vi "Move piezo.vi"(7 "error in (no error)":errorcluster, 8 "MOVE TO [MICRON]":dbl=1.0 format="%0.2f", 9 "notifier out":refnum<notifier>, 10 "Hardware Config In":T1={"physical channels"="Dev4/ao0", "MAX   VOLTAGE"=10.0, "MIN   VOLTAGE"=0.0}) -> (0 "error out":errorcluster, 3 "Hardware Config Out":T1={"physical channels"="Dev4/ao0", "MAX   VOLTAGE"=10.0, "MIN   VOLTAGE"=0.0})   [LabVIEW 2013, in "Piezo.lvlib"]
uses:
  Piezo/Piezo.lvlib
  Piezo/Piezo display.ctl
  Untitled Project 3 Andrea/piezo new/Hardware Configuration Piezo out.ctl
  <vilib>/DAQmx/write.llb/DAQmx Write (Analog DBL 1Chan 1Samp).vi
  <vilib>/DAQmx/create/channels.llb/DAQmx Create Channel (AO-Voltage-Basic).vi
  <vilib>/DAQmx/miscellaneous.llb/DAQmx Fill In Error Info.vi
panel:
  out "PiezoPosition":sgl
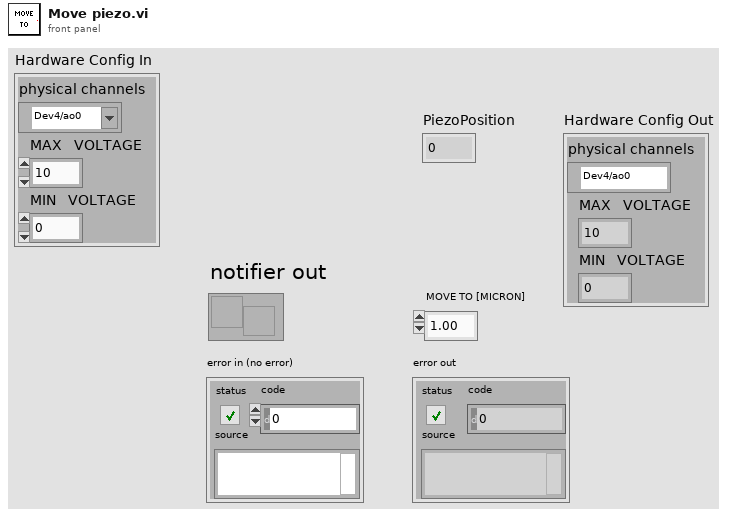
[diagram p1: front panel]
types:
  T1 = typedef "Hardware Configuration Piezo out.ctl" = cluster{"physical channels":tag, "MAX   VOLTAGE":dbl, "MIN   VOLTAGE":dbl}
  T2 = typedef "Piezo.lvlib/Piezo display.ctl" = cluster{"PiezoPosition":sgl, "Counter Time":i32}
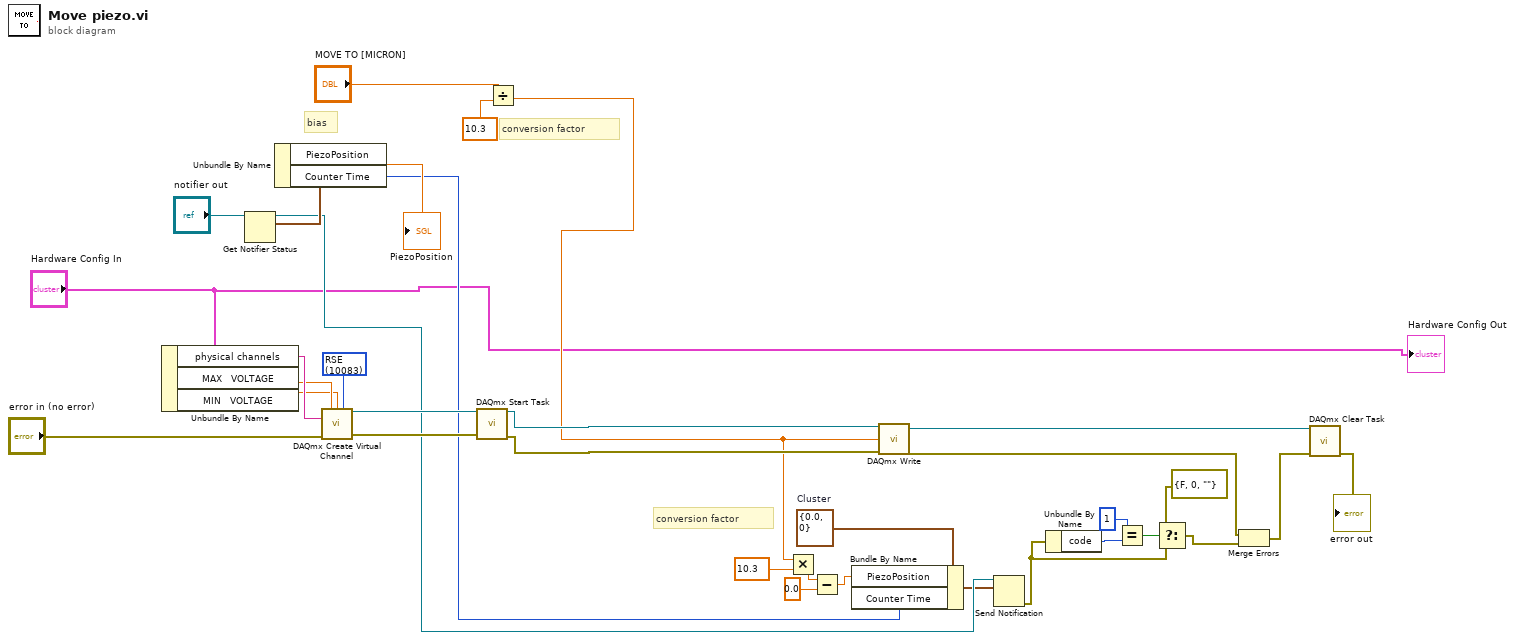
[diagram p0: block diagram]
diagram:
  w14 = T2 {"PiezoPosition"=0.0, "Counter Time"=0}  # Cluster
  w30 = 10083 items=["Default"=-1, "RSE"=10083, "Differential"=10106, "Pseudodifferential"=12529] ("output terminal configuration")
  # "conversion factor"
  # "bias"
  # "conversion factor"
  n1 = Unbundle By Name("Hardware Config In") -> ("physical channels"=w27:tag, "MAX   VOLTAGE"=w26:dbl, "MIN   VOLTAGE"=w25:dbl)
  n2 = Get Notifier Status(notifier="notifier out") -> (notifier out=w18:refnum<notifier>, current notification=w32:T2)  [unwired: 1 in, 3 out]
  n3 = Unbundle By Name(w32) -> ("PiezoPosition"=→"PiezoPosition":sgl, "Counter Time"=w17:i32)
  n4 = call-poly <vilib>:"DAQmx Create Virtual Channel.vi"("maximum value"=w26, "minimum value"=w25, "output terminal configuration"=w30, "physical channels"=w27, "error in"="error in (no error)") -> ("task out"=w29:refnum<k21>, "error out"=w28:errorcluster)  [unwired: 9 in]
  n5 = call <vilib>:"DAQmx Start Task.vi"("task/channels in"=w29, "error in"=w28) -> ("task out"=w21:refnum<k21>, "error out"=w20:errorcluster)  [unwired: 12 in]
  n6 = Divide(x="MOVE TO [MICRON]", y=10.3) -> (x/y=w2:dbl)
  n7 = Multiply(x=w2, y=10.3) -> (x*y=w4:dbl)
  n8 = Subtract(x=w4, y=0.0) -> (x-y=w5:dbl)
  n9 = Bundle By Name(cluster=w14, "PiezoPosition"=w5, "Counter Time"=w17) -> (w15:T2)
  n10 = call-poly <vilib>:"DAQmx Write.vi"("task/channels in"=w21, "data"=w2, "error in"=w20) -> ("task out"=w23:refnum<k21>, "error out"=w9:errorcluster)  [unwired: 10 in, 1 out]
  n11 = Send Notification(notification=w15, notifier=w18) -> (error out=w8:errorcluster)  [unwired: 1 in, 1 out]
  n12 = Unbundle By Name(w8) -> ("code"=w13:i32)
  n13 = Equal?(x=1, y=w13) -> (x = y?=w11:bool)
  n14 = Select(t=errorcluster {"status"=FALSE, "code"=0, "source"=""} ("error constant"), s=w11, f=w8) -> (s? t:f=w7:errorcluster)
  n15 = Merge Errors(w9, w7) -> (w22:errorcluster)
  n16 = call <vilib>:"DAQmx Clear Task.vi"("task in"=w23, "error in"=w22) -> ("error out"=→"error out":errorcluster)  [unwired: 13 in]
  "Hardware Config Out" <- "Hardware Config In"
